vi "Set Stability Mode.vi"(2 "error in":T1, 3 "Stability Mode":u16(ring) items=["Auto", "Manual", "Test"], 4 "connection ID":refnum<visa-resource-name>) -> (0 "error out":T1, 1 "connection ID out":refnum<visa-resource-name>)   [LabVIEW 2019]
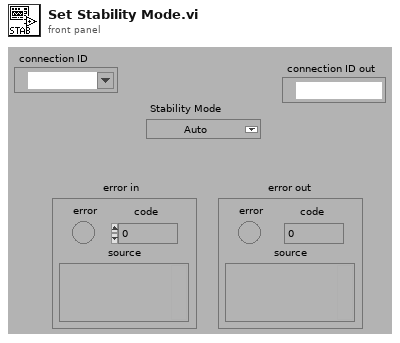
[diagram p1: front panel]
types:
  T1 = cluster{"error":bool, "code":i32, "source":string}
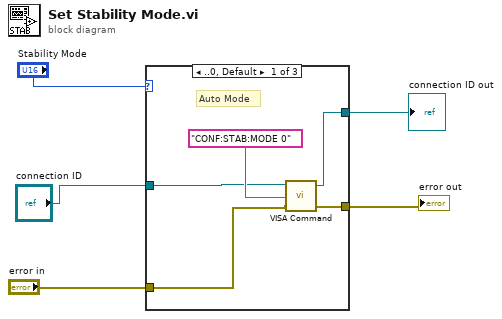
[diagram p0: block diagram]
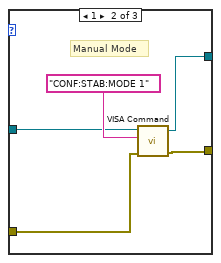
[diagram p2: hidden frame]
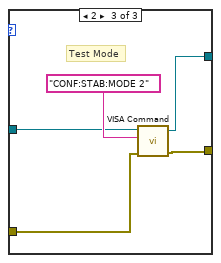
[diagram p3: hidden frame]
diagram:
  n1 = case shown="..0, Default" "Stability Mode" {
    tunnel: "error in" -> [w9 w14 w19]
    tunnel: [w8 w13 w18] -> w3
    tunnel: "connection ID" -> [w7 w12 w17]
    tunnel: [w6 w11 w16] -> w1
    frame ..0, Default {
      # "Auto Mode"
      n2 = call "VISA Command.vi"("error in (no error)"=w9, "Command"="CONF:STAB:MODE 0", "VISA resource name"=w7) -> ("error out"=w8:errorcluster, "VISA resource name out"=w6:refnum<visa-resource-name>)  [unwired: 1 in, 1 out]
    }
    frame 1 {
      # "Manual Mode"
      n3 = call "VISA Command.vi"("error in (no error)"=w14, "Command"="CONF:STAB:MODE 1", "VISA resource name"=w12) -> ("error out"=w13:errorcluster, "VISA resource name out"=w11:refnum<visa-resource-name>)  [unwired: 1 in, 1 out]
    }
    frame 2 {
      # "Test Mode"
      n4 = call "VISA Command.vi"("error in (no error)"=w19, "Command"="CONF:STAB:MODE 2", "VISA resource name"=w17) -> ("error out"=w18:errorcluster, "VISA resource name out"=w16:refnum<visa-resource-name>)  [unwired: 1 in, 1 out]
    }
  }
  "error out" <- w3
  "connection ID out" <- w1
